vi "add.vi"() -> ()   [LabVIEW 2025]
uses:
  ArrayIncMSVC/ArrayInc/x64/Release/ArrayInc.dll
panel:
  out "x-y 2":dbl
  out "sum 2":u8
  out "sum":u8
  out "x-y":dbl
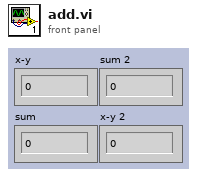
[diagram p1: front panel]
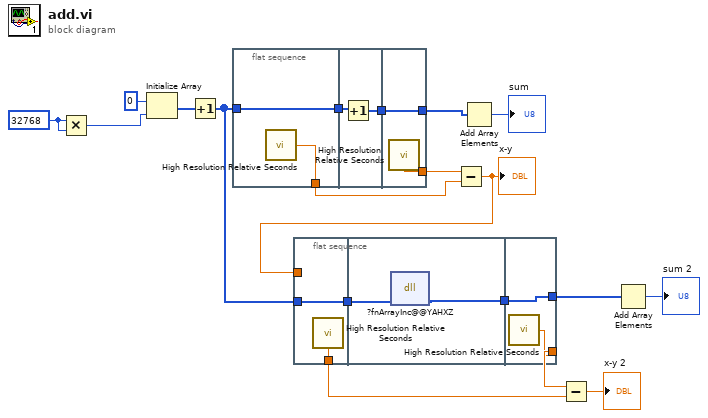
[diagram p0: block diagram]
diagram:
  w18 = 32768 ("x")
  n1 = Multiply(x=w18, y=w18) -> (x*y=w17:i32)
  n2 = Initialize Array(u8 0 ("element"), w17) -> (w16:u8[])
  n3 = Increment(x=w16) -> (x+1=w9:u8[])
  n4 = flat-sequence {
    tunnel: w9 -> [w21]
    tunnel: [w21] -> w15
    tunnel: [w20] -> w12
    tunnel: w15 -> [w23]
    tunnel: [w22] -> w14
    tunnel: w14 -> [w25]
    tunnel: [w25] -> w11
    tunnel: [w24] -> w13
    frame #0 {
      n5 = call <vilib>:"High Resolution Relative Seconds.vi"() -> ("relative seconds"=w20:dbl)
    }
    frame #1 {
      n6 = Increment(x=w23) -> (x+1=w22:u8[])
    }
    frame #2 {
      n7 = call <vilib>:"High Resolution Relative Seconds.vi"() -> ("relative seconds"=w24:dbl)
    }
  }
  n8 = flat-sequence {
    tunnel: w9 -> [w27]
    tunnel: [w27] -> w8
    tunnel: [w26] -> w2
    tunnel: w1 -> [_]
    tunnel: w8 -> [w29]
    tunnel: [w28] -> w5
    tunnel: [w31] -> w6
    tunnel: w5 -> [w31]
    tunnel: [w30] -> w3
    frame #0 {
      n9 = call <vilib>:"High Resolution Relative Seconds.vi"() -> ("relative seconds"=w26:dbl)
    }
    frame #1 {
      n10 = dll-call lib="C:/Users/Andrey/Desktop/ArrayIncMSVC/ArrayInc/x64/Release/ArrayInc.dll" fn="?fnArrayInc@@YAHXZ"("array"=w29) -> ("array"=w28:u8[])  [unwired: 4 in, 2 out]
    }
    frame #2 {
      n11 = call <vilib>:"High Resolution Relative Seconds.vi"() -> ("relative seconds"=w30:dbl)
    }
  }
  n12 = Subtract(x=w13, y=w12) -> (x-y=w1:dbl)
  "x-y" <- w1
  n13 = Add Array Elements(numeric array=w11) -> (sum=→"sum":u8)
  n14 = Subtract(x=w3, y=w2) -> (x-y=→"x-y 2":dbl)
  n15 = Add Array Elements(numeric array=w6) -> (sum=→"sum 2":u8)
